vi "RX OOB Test Cases.vi"() -> (0 "error out":errorcluster, 2 "status":string, 3 "pass":bool)   [LabVIEW 2021]
uses:
  OOB_Rx/CIFCoreOOB_Rx.lvclass/CIFCoreOOB_Rx.ctl
  CIFUtilities/CIFOutOfBand/CIFOutOfBand.lvclass/CIFOutOfBand.ctl
  OOB_Rx/Typedef/OOB Core Commands.ctl
  OOB_Rx/Typedef/Channel Connection Data.ctl
  OOB_Rx/Private/Command Settings.vi
  CIFUtilities/CIFOutOfBand/Accessors/Write Local OOB Data.vi
  CIFUtilities/CIFOutOfBand/Write OOB DVR.vi
  CIFUtilities/CIFOutOfBand/Utilities/Command to Bitwise Command.vi
  CIFUtilities/CIFOutOfBand/Read OOB DVR.vi
  OOB_Rx/Private/Read Payload.vi
  OOB_Rx/CIFCoreOOB_Rx.lvclass
  D:/dev/CIF-LVCore/src/CIFUtilities/CIFOutOfBand/CIFOutOfBand.lvclass
  CIFUtilities/CIFOutOfBand/Init OOB.vi
  <vilib>/addons/_JKI.lib/Serialization/JSON/Library/Unflatten From JSON String.vi
  <vilib>/addons/_JKI.lib/Serialization/JSON/JKI JSON Serialization.lvlib
  CIFUtilities/CIFOutOfBand/CIFOutOfBand.lvclass
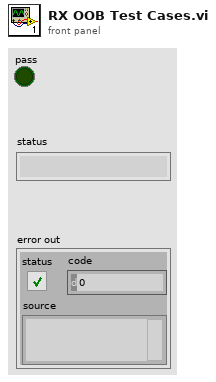
[diagram p1: front panel]
types:
  T1 = cluster{"Numeric":dbl, "Array":cluster{"Numeric":dbl, "String":string, "Boolean":bool}[], "string":string, "Null array":u8[]}
  T2 = typedef "CIFCoreOOB_Rx.lvclass/OOB Core Commands.ctl" = enum8{"Start", "Pause", "Stop", "RefreshStats", "UpdateConfig", "Connect Channel"}
  T3 = typedef "CIFCoreOOB_Rx.lvclass/Channel Connection Data.ctl" = cluster{"Publisher Name":string, "Subscriber Name":string, "Connection Data":variant}
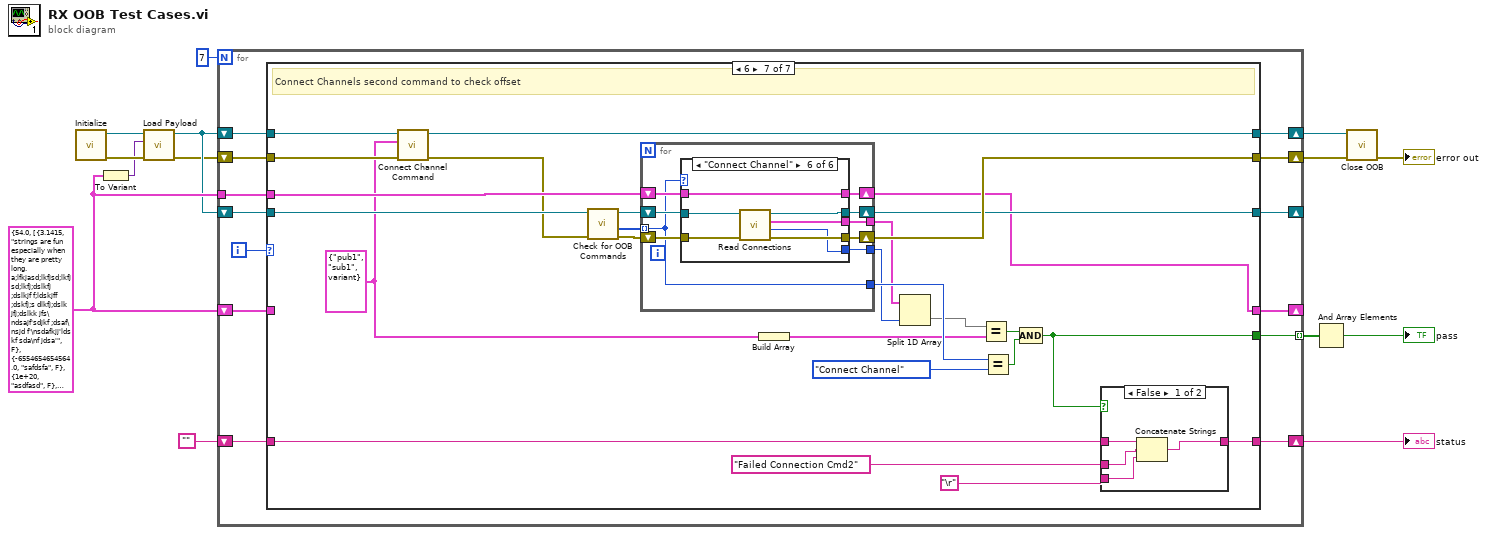
[diagram p0: block diagram]
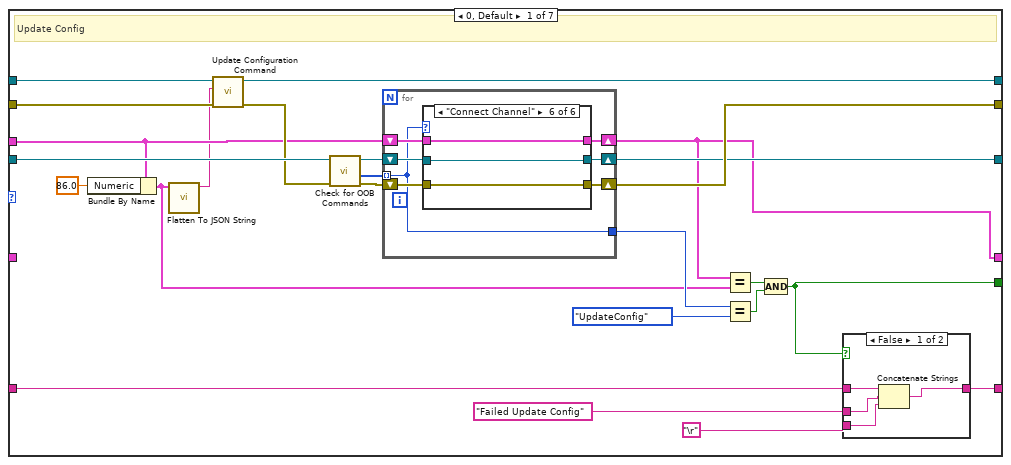
[diagram p2: hidden frame]
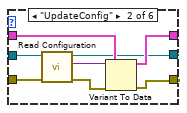
[diagram p4: hidden frame]
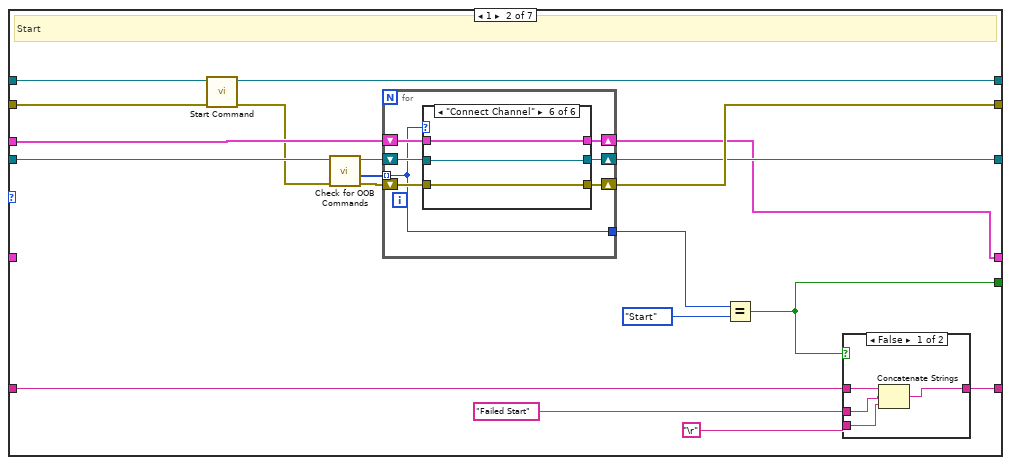
[diagram p9: hidden frame]
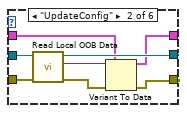
[diagram p11: hidden frame]
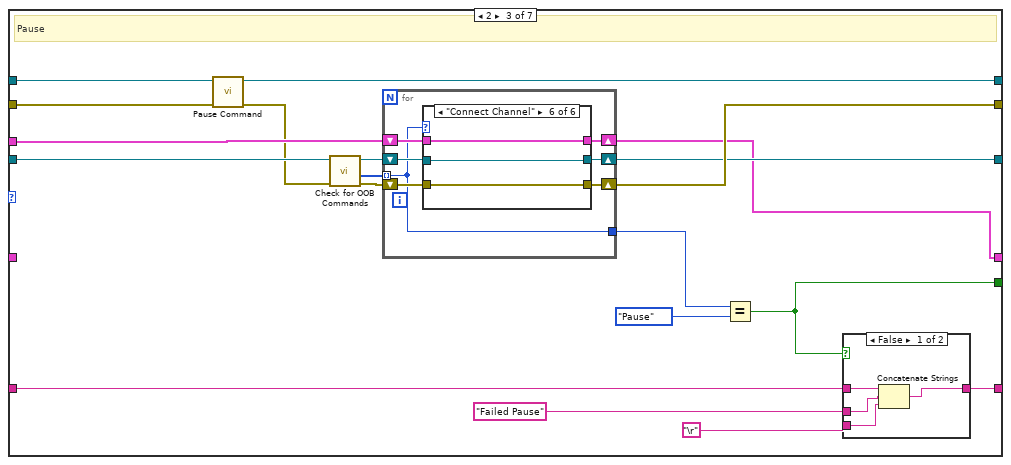
[diagram p16: hidden frame]
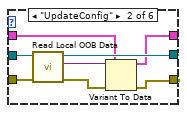
[diagram p18: hidden frame]
diagram:
  w14 = T1 {"Numeric"=54.0, "Array"=[{"Numeric"=3.1415, "String"="strings are fun especially when they are pretty long. a;lfkjasd;lkfjsd;lkfjsd;lkfj;dslkfj ;dslkjf f;ldskjff ;dskfj;s dlkfj;dslk jfj;dslkk jfs\ndsajf'sdjkf ;dsaf\nsjd f'\nsdafkjj'lds kf sda\nf jdsa'", "Boolean"=FALSE}, {"Numeric"=-6554654654564.0, "String"="safdsfa", "Boolean"=FALSE}, {"Numeric"=1e+20, "String"="asdfasd", "Boolean"=FALSE}, {"Numeric"=2.0, "String"="afd", "Boolean"=TRUE}, {"Numeric"=12.34, "String"="data", "Boolean"=FALSE}], "string"="strings", "Null array"=[0]} ("Test Config")
  n1 = call "Initialize.vi"() -> ("error out"=w7:errorcluster, "CoreOOB_Rx out"=w6:refnum<class "CIFCoreOOB_Rx.lvclass">)  [unwired: 10 in]
  n2 = To Variant(anything=w14) -> (Variant=w3:variant)
  n3 = call "Load Payload.vi"("error in (no error)"=w7, "Configuration Payload"=w3, "CoreOOB_Rx in"=w6) -> ("error out"=w4:errorcluster, "CoreOOB_Rx out"=w5:refnum<class "CIFCoreOOB_Rx.lvclass">)  [unwired: 7 in]
  n4 = for {
    N: 7 -> [_]
    tunnel: [w27] -> w11 mode=indexing
    tunnel: w14 -> [w25]
    shift-right: [w23] -> w12
    shift-left: w4 -> [w26]
    shift-right: [w21] -> w13
    shift-left: w5 -> [w24]
    shift-right: [w19] -> _
    shift-left: w5 -> [w20]
    shift-right: [w18] -> _
    shift-left: w14 -> [w17]
    shift-right: [w15] -> w8
    shift-left: "" -> [w16]
    i -> [w22]
    n5 = case shown="6" w22 {
      tunnel: [w39 w87 w141 w199 w253 w303 w370] -> w27
      tunnel: w26 -> [w34 w96 w144 w197 w251 w313 w380]
      tunnel: w25 -> [w32 w105 w159 w213 w267 w328 w395]
      tunnel: w24 -> [w36 w97 w145 w198 w252 w314 w381]
      tunnel: [w51 w104 w158 w212 w266 w327 w394] -> w23
      tunnel: [w35 w95 w142 w195 w249 w311 w378] -> w21
      tunnel: w20 -> [w45 w94 w151 w205 w259 w320 w387]
      tunnel: [w50 w103 w157 w211 w265 w326 w393] -> w19
      tunnel: [w28 w102 w156 w210 w264 w325 w392] -> w18
      tunnel: w17 -> [_ _ _ _ _ _ _]
      tunnel: w16 -> [w49 w101 w155 w209 w263 w324 w391]
      tunnel: [w48 w100 w154 w208 w262 w323 w390] -> w15
      frame 0, Default {
        # "Update Config"
        n6 = Bundle By Name(cluster=w32, "Numeric"=86.0) -> (w29:T1)
        n7 = call <vilib>:"Flatten To JSON String.vi"("Variant"=w29) -> ("JSON String"=w30:string)  [unwired: 9 in, 1 out]
        n8 = call "Update Configuration Command.vi"("error in"=w34, "Config JSON"=w30, "CoreOOB_Rx in"=w36) -> ("error out"=w33:errorcluster, "CoreOOB_Rx out"=w35:refnum<class "CIFCoreOOB_Rx.lvclass">)  [unwired: 7 in]
        n9 = call "Check for OOB Commands.vi"("error in (no error)"=w33, "CoreOOB_Rx in"=w45) -> ("error out"=w44:errorcluster, "Commands"=w42:T2[], "CoreOOB_Rx out"=w43:refnum<class "CIFCoreOOB_Rx.lvclass">)  [unwired: 6 in, 1 out]
        n10 = for {
          tunnel: w42 -> [w52] mode=indexing
          shift-right: [w53] -> w28
          shift-left: w32 -> [w58]
          shift-right: [w57] -> w51
          shift-left: w44 -> [w55]
          shift-right: [w56] -> w50
          shift-left: w43 -> [w54]
          tunnel: [w52] -> w38
          n11 = case shown="\"Connect Channel\"" w52 {
            tunnel: w54 -> [w60 w65 w71 w74 w77 w80]
            tunnel: w55 -> [w59 w66 w70 w73 w78 w81]
            tunnel: [w60 w64 w71 w74 w77 w80] -> w56
            tunnel: w58 -> [w61 w69 w72 w75 w76 w79]
            tunnel: [w59 w68 w70 w73 w78 w81] -> w57
            tunnel: [w61 w67 w72 w75 w76 w79] -> w53
            frame "Start" {
            }
            frame "UpdateConfig" {
              n12 = call "Read Configuration.vi"("error in"=w66, "CoreOOB_Rx in"=w65) -> ("error out"=w62:errorcluster, "Configuration Data"=w63:variant, "CoreOOB_Rx out"=w64:refnum<class "CIFCoreOOB_Rx.lvclass">)  [unwired: 7 in]
              n13 = Variant To Data(error in=w62, type=w69, Variant=w63) -> (data=w67:T1, error out=w68:errorcluster)
            }
            frame "Pause" {
            }
            frame "Stop" {
            }
            frame "RefreshStats" {
            }
            frame "Connect Channel" {
            }
          }
        }
        n14 = Equal?(x=w28, y=w29) -> (x = y?=w41:bool)
        n15 = Equal?(x=w38, y=OOB_Core_Commands."UpdateConfig") -> (x = y?=w40:bool)
        n16 = Compound Arithmetic op=AND(w41, w40) -> (w39:bool)
        n17 = case shown="False" w39 {
          tunnel: w49 -> [w85 w86]
          tunnel: [w82 w86] -> w48
          tunnel: "Failed Update Config" -> [w84 _]
          tunnel: "\r" -> [w83 _]
          frame False {
            n18 = Concatenate Strings(w85, w84, w83) -> (w82:string)
          }
          frame True {
          }
        }
      }
      frame 1 {
        # "Start"
        n19 = call "Start Command.vi"("error in"=w96, "CoreOOB_Rx in"=w97) -> ("error out"=w93:errorcluster, "CoreOOB_Rx out"=w95:refnum<class "CIFCoreOOB_Rx.lvclass">)  [unwired: 8 in]
        n20 = call "Check for OOB Commands.vi"("error in (no error)"=w93, "CoreOOB_Rx in"=w94) -> ("error out"=w92:errorcluster, "Commands"=w90:T2[], "CoreOOB_Rx out"=w91:refnum<class "CIFCoreOOB_Rx.lvclass">)  [unwired: 6 in, 1 out]
        n21 = for {
          tunnel: w90 -> [w106] mode=indexing
          shift-right: [w107] -> w102
          shift-left: w105 -> [w112]
          shift-right: [w111] -> w104
          shift-left: w92 -> [w109]
          shift-right: [w110] -> w103
          shift-left: w91 -> [w108]
          tunnel: [w106] -> w89
          n22 = case shown="\"Connect Channel\"" w106 {
            tunnel: w108 -> [w113 w123 w125 w128 w131 w134]
            tunnel: w109 -> [w114 w122 w124 w127 w132 w135]
            tunnel: [w113 w120 w125 w128 w131 w134] -> w110
            tunnel: w112 -> [w115 w118 w126 w129 w130 w133]
            tunnel: [w114 w117 w124 w127 w132 w135] -> w111
            tunnel: [w115 w116 w126 w129 w130 w133] -> w107
            frame "Start" {
            }
            frame "UpdateConfig" {
              n23 = call "Read Local OOB Data.vi"("error in"=w122, "OOB in"=w123) -> ("error out"=w121:errorcluster, "Local OOB Data"=w119:variant, "OOB out"=w120:refnum<class "CIFCoreOOB_Rx.lvclass">)  [unwired: 7 in]
              n24 = Variant To Data(error in=w121, type=w118, Variant=w119) -> (data=w116:T1, error out=w117:errorcluster)
            }
            frame "Pause" {
            }
            frame "Stop" {
            }
            frame "RefreshStats" {
            }
            frame "Connect Channel" {
            }
          }
        }
        n25 = Equal?(x=w89, y=OOB_Core_Commands."Start") -> (x = y?=w87:bool)
        n26 = case shown="False" w87 {
          tunnel: w101 -> [w139 w140]
          tunnel: [w136 w140] -> w100
          tunnel: "Failed Start" -> [w138 _]
          tunnel: "\r" -> [w137 _]
          frame False {
            n27 = Concatenate Strings(w139, w138, w137) -> (w136:string)
          }
          frame True {
          }
        }
      }
      frame 2 {
        # "Pause"
        n28 = call "Pause Command.vi"("error in"=w144, "CoreOOB_Rx in"=w145) -> ("error out"=w143:errorcluster, "CoreOOB_Rx out"=w142:refnum<class "CIFCoreOOB_Rx.lvclass">)  [unwired: 8 in]
        n29 = call "Check for OOB Commands.vi"("error in (no error)"=w143, "CoreOOB_Rx in"=w151) -> ("error out"=w150:errorcluster, "Commands"=w148:T2[], "CoreOOB_Rx out"=w149:refnum<class "CIFCoreOOB_Rx.lvclass">)  [unwired: 6 in, 1 out]
        n30 = for {
          tunnel: w148 -> [w160] mode=indexing
          shift-right: [w161] -> w156
          shift-left: w159 -> [w166]
          shift-right: [w165] -> w158
          shift-left: w150 -> [w163]
          shift-right: [w164] -> w157
          shift-left: w149 -> [w162]
          tunnel: [w160] -> w147
          n31 = case shown="\"Connect Channel\"" w160 {
            tunnel: w162 -> [w168 w177 w179 w182 w185 w188]
            tunnel: w163 -> [w167 w176 w178 w181 w186 w189]
            tunnel: [w168 w174 w179 w182 w185 w188] -> w164
            tunnel: w166 -> [w169 w172 w180 w183 w184 w187]
            tunnel: [w167 w171 w178 w181 w186 w189] -> w165
            tunnel: [w169 w170 w180 w183 w184 w187] -> w161
            frame "Start" {
            }
            frame "UpdateConfig" {
              n32 = call "Read Local OOB Data.vi"("error in"=w176, "OOB in"=w177) -> ("error out"=w175:errorcluster, "Local OOB Data"=w173:variant, "OOB out"=w174:refnum<class "CIFCoreOOB_Rx.lvclass">)  [unwired: 7 in]
              n33 = Variant To Data(error in=w175, type=w172, Variant=w173) -> (data=w170:T1, error out=w171:errorcluster)
            }
            frame "Pause" {
            }
            frame "Stop" {
            }
            frame "RefreshStats" {
            }
            frame "Connect Channel" {
            }
          }
        }
        n34 = Equal?(x=w147, y=OOB_Core_Commands."Pause") -> (x = y?=w141:bool)
        n35 = case shown="False" w141 {
          tunnel: w155 -> [w193 w194]
          tunnel: [w190 w194] -> w154
          tunnel: "Failed Pause" -> [w192 _]
          tunnel: "\r" -> [w191 _]
          frame False {
            n36 = Concatenate Strings(w193, w192, w191) -> (w190:string)
          }
          frame True {
          }
        }
      }
      frame 3 {
        # "Stop"
        n37 = call "Stop Command.vi"("error in"=w197, "CoreOOB_Rx in"=w198) -> ("error out"=w196:errorcluster, "CoreOOB_Rx out"=w195:refnum<class "CIFCoreOOB_Rx.lvclass">)  [unwired: 8 in]
        n38 = call "Check for OOB Commands.vi"("error in (no error)"=w196, "CoreOOB_Rx in"=w205) -> ("error out"=w204:errorcluster, "Commands"=w202:T2[], "CoreOOB_Rx out"=w203:refnum<class "CIFCoreOOB_Rx.lvclass">)  [unwired: 6 in, 1 out]
        n39 = for {
          tunnel: w202 -> [w214] mode=indexing
          shift-right: [w215] -> w210
          shift-left: w213 -> [w220]
          shift-right: [w219] -> w212
          shift-left: w204 -> [w217]
          shift-right: [w218] -> w211
          shift-left: w203 -> [w216]
          tunnel: [w214] -> w201
          n40 = case shown="\"Connect Channel\"" w214 {
            tunnel: w216 -> [w222 w231 w233 w236 w239 w242]
            tunnel: w217 -> [w221 w230 w232 w235 w240 w243]
            tunnel: [w222 w228 w233 w236 w239 w242] -> w218
            tunnel: w220 -> [w223 w226 w234 w237 w238 w241]
            tunnel: [w221 w225 w232 w235 w240 w243] -> w219
            tunnel: [w223 w224 w234 w237 w238 w241] -> w215
            frame "Start" {
            }
            frame "UpdateConfig" {
              n41 = call "Read Local OOB Data.vi"("error in"=w230, "OOB in"=w231) -> ("error out"=w229:errorcluster, "Local OOB Data"=w227:variant, "OOB out"=w228:refnum<class "CIFCoreOOB_Rx.lvclass">)  [unwired: 7 in]
              n42 = Variant To Data(error in=w229, type=w226, Variant=w227) -> (data=w224:T1, error out=w225:errorcluster)
            }
            frame "Pause" {
            }
            frame "Stop" {
            }
            frame "RefreshStats" {
            }
            frame "Connect Channel" {
            }
          }
        }
        n43 = Equal?(x=w201, y=OOB_Core_Commands."Stop") -> (x = y?=w199:bool)
        n44 = case shown="False" w199 {
          tunnel: w209 -> [w247 w248]
          tunnel: [w244 w248] -> w208
          tunnel: "Failed Stop" -> [w246 _]
          tunnel: "\r" -> [w245 _]
          frame False {
            n45 = Concatenate Strings(w247, w246, w245) -> (w244:string)
          }
          frame True {
          }
        }
      }
      frame 4 {
        # "Refresh"
        n46 = call "Refresh Stats Command.vi"("error in"=w251, "CoreOOB_Rx in"=w252) -> ("error out"=w250:errorcluster, "CoreOOB_Rx out"=w249:refnum<class "CIFCoreOOB_Rx.lvclass">)  [unwired: 8 in]
        n47 = call "Check for OOB Commands.vi"("error in (no error)"=w250, "CoreOOB_Rx in"=w259) -> ("error out"=w258:errorcluster, "Commands"=w256:T2[], "CoreOOB_Rx out"=w257:refnum<class "CIFCoreOOB_Rx.lvclass">)  [unwired: 6 in, 1 out]
        n48 = for {
          tunnel: w256 -> [w268] mode=indexing
          shift-right: [w269] -> w264
          shift-left: w267 -> [w274]
          shift-right: [w273] -> w266
          shift-left: w258 -> [w271]
          shift-right: [w272] -> w265
          shift-left: w257 -> [w270]
          tunnel: [w268] -> w255
          n49 = case shown="\"Connect Channel\"" w268 {
            tunnel: w270 -> [w276 w285 w287 w290 w293 w296]
            tunnel: w271 -> [w275 w284 w286 w289 w294 w297]
            tunnel: [w276 w282 w287 w290 w293 w296] -> w272
            tunnel: w274 -> [w277 w280 w288 w291 w292 w295]
            tunnel: [w275 w279 w286 w289 w294 w297] -> w273
            tunnel: [w277 w278 w288 w291 w292 w295] -> w269
            frame "Start" {
            }
            frame "UpdateConfig" {
              n50 = call "Read Local OOB Data.vi"("error in"=w284, "OOB in"=w285) -> ("error out"=w283:errorcluster, "Local OOB Data"=w281:variant, "OOB out"=w282:refnum<class "CIFCoreOOB_Rx.lvclass">)  [unwired: 7 in]
              n51 = Variant To Data(error in=w283, type=w280, Variant=w281) -> (data=w278:T1, error out=w279:errorcluster)
            }
            frame "Pause" {
            }
            frame "Stop" {
            }
            frame "RefreshStats" {
            }
            frame "Connect Channel" {
            }
          }
        }
        n52 = Equal?(x=w255, y=OOB_Core_Commands."RefreshStats") -> (x = y?=w253:bool)
        n53 = case shown="False" w253 {
          tunnel: w263 -> [w301 w302]
          tunnel: [w298 w302] -> w262
          tunnel: "Failed Refresh" -> [w300 _]
          tunnel: "\r" -> [w299 _]
          frame False {
            n54 = Concatenate Strings(w301, w300, w299) -> (w298:string)
          }
          frame True {
          }
        }
      }
      frame 5 {
        w307 = T3 {"Publisher Name"="pub", "Subscriber Name"="sub", "Connection Data"=variant} ("Channel Connection Data")
        # "Connect Channels"
        n55 = call "Connect Channel Command.vi"("error in"=w313, "Channel Connection Data"=w307, "CoreOOB_Rx in"=w314) -> ("error out"=w312:errorcluster, "CoreOOB_Rx out"=w311:refnum<class "CIFCoreOOB_Rx.lvclass">)  [unwired: 7 in]
        n56 = call "Check for OOB Commands.vi"("error in (no error)"=w312, "CoreOOB_Rx in"=w320) -> ("error out"=w319:errorcluster, "Commands"=w317:T2[], "CoreOOB_Rx out"=w318:refnum<class "CIFCoreOOB_Rx.lvclass">)  [unwired: 6 in, 1 out]
        n57 = for {
          tunnel: w317 -> [w331] mode=indexing
          shift-right: [w332] -> w325
          shift-left: w328 -> [w337]
          shift-right: [w336] -> w327
          shift-left: w319 -> [w334]
          shift-right: [w335] -> w326
          shift-left: w318 -> [w333]
          tunnel: [w331] -> w316
          tunnel: [w330] -> w310
          tunnel: [w329] -> w309
          n58 = case shown="\"Connect Channel\"" w331 {
            tunnel: w333 -> [w339 w348 w350 w353 w356 w363]
            tunnel: w334 -> [w338 w347 w349 w352 w357 w362]
            tunnel: [w339 w345 w350 w353 w356 w361] -> w335
            tunnel: w337 -> [w340 w343 w351 w354 w355 w364]
            tunnel: [w338 w342 w349 w352 w357 w360] -> w336
            tunnel: [w340 w341 w351 w354 w355 w364] -> w332
            tunnel: [_ _ _ _ _ w359] -> w330
            tunnel: [_ _ _ _ _ w358] -> w329
            frame "Start" {
            }
            frame "UpdateConfig" {
              n59 = call "Read Local OOB Data.vi"("error in"=w347, "OOB in"=w348) -> ("error out"=w346:errorcluster, "Local OOB Data"=w344:variant, "OOB out"=w345:refnum<class "CIFCoreOOB_Rx.lvclass">)  [unwired: 7 in]
              n60 = Variant To Data(error in=w346, type=w343, Variant=w344) -> (data=w341:T1, error out=w342:errorcluster)
            }
            frame "Pause" {
            }
            frame "Stop" {
            }
            frame "RefreshStats" {
            }
            frame "Connect Channel" {
              n61 = call "Read Connections.vi"("error in"=w362, "CoreOOB_Rx in"=w363) -> ("error out"=w360:errorcluster, "Offset"=w358:i32, "Connections"=w359:T3[], "CoreOOB_Rx out"=w361:refnum<class "CIFCoreOOB_Rx.lvclass">)  [unwired: 6 in]
            }
          }
        }
        n62 = Build Array(w307) -> (w306:T3[])
        n63 = Split 1D Array(array=w310, index=w309) -> (second subarray=w308:T3[])  [unwired: 1 out]
        n64 = Equal?(x=w308, y=w306) -> (x = y?=w305:bool)
        n65 = Equal?(x=w316, y=OOB_Core_Commands."Connect Channel") -> (x = y?=w304:bool)
        n66 = Compound Arithmetic op=AND(w305, w304) -> (w303:bool)
        n67 = case shown="False" w303 {
          tunnel: w324 -> [w368 w369]
          tunnel: [w365 w369] -> w323
          tunnel: "Failed Connection Cmd1" -> [w367 _]
          tunnel: "\r" -> [w366 _]
          frame False {
            n68 = Concatenate Strings(w368, w367, w366) -> (w365:string)
          }
          frame True {
          }
        }
      }
      frame 6 {
        w374 = T3 {"Publisher Name"="pub1", "Subscriber Name"="sub1", "Connection Data"=variant} ("Channel Connection Data")
        # "Connect Channels second command to check offset"
        n69 = call "Connect Channel Command.vi"("error in"=w380, "Channel Connection Data"=w374, "CoreOOB_Rx in"=w381) -> ("error out"=w379:errorcluster, "CoreOOB_Rx out"=w378:refnum<class "CIFCoreOOB_Rx.lvclass">)  [unwired: 7 in]
        n70 = call "Check for OOB Commands.vi"("error in (no error)"=w379, "CoreOOB_Rx in"=w387) -> ("error out"=w386:errorcluster, "Commands"=w384:T2[], "CoreOOB_Rx out"=w385:refnum<class "CIFCoreOOB_Rx.lvclass">)  [unwired: 6 in, 1 out]
        n71 = for {
          tunnel: w384 -> [w398] mode=indexing
          shift-right: [w399] -> w392
          shift-left: w395 -> [w404]
          shift-right: [w403] -> w394
          shift-left: w386 -> [w401]
          shift-right: [w402] -> w393
          shift-left: w385 -> [w400]
          tunnel: [w398] -> w383
          tunnel: [w397] -> w377
          tunnel: [w396] -> w376
          n72 = case shown="\"Connect Channel\"" w398 {
            tunnel: w400 -> [w406 w415 w417 w420 w423 w430]
            tunnel: w401 -> [w405 w414 w416 w419 w424 w429]
            tunnel: [w406 w412 w417 w420 w423 w428] -> w402
            tunnel: w404 -> [w407 w410 w418 w421 w422 w431]
            tunnel: [w405 w409 w416 w419 w424 w427] -> w403
            tunnel: [w407 w408 w418 w421 w422 w431] -> w399
            tunnel: [_ _ _ _ _ w426] -> w397
            tunnel: [_ _ _ _ _ w425] -> w396
            frame "Start" {
            }
            frame "UpdateConfig" {
              n73 = call "Read Local OOB Data.vi"("error in"=w414, "OOB in"=w415) -> ("error out"=w413:errorcluster, "Local OOB Data"=w411:variant, "OOB out"=w412:refnum<class "CIFCoreOOB_Rx.lvclass">)  [unwired: 7 in]
              n74 = Variant To Data(error in=w413, type=w410, Variant=w411) -> (data=w408:T1, error out=w409:errorcluster)
            }
            frame "Pause" {
            }
            frame "Stop" {
            }
            frame "RefreshStats" {
            }
            frame "Connect Channel" {
              n75 = call "Read Connections.vi"("error in"=w429, "CoreOOB_Rx in"=w430) -> ("error out"=w427:errorcluster, "Offset"=w425:i32, "Connections"=w426:T3[], "CoreOOB_Rx out"=w428:refnum<class "CIFCoreOOB_Rx.lvclass">)  [unwired: 6 in]
            }
          }
        }
        n76 = Build Array(w374) -> (w373:T3[])
        n77 = Split 1D Array(array=w377, index=w376) -> (second subarray=w375:T3[])  [unwired: 1 out]
        n78 = Equal?(x=w375, y=w373) -> (x = y?=w372:bool)
        n79 = Equal?(x=w383, y=OOB_Core_Commands."Connect Channel") -> (x = y?=w371:bool)
        n80 = Compound Arithmetic op=AND(w372, w371) -> (w370:bool)
        n81 = case shown="False" w370 {
          tunnel: w391 -> [w435 w436]
          tunnel: [w432 w436] -> w390
          tunnel: "Failed Connection Cmd2" -> [w434 _]
          tunnel: "\r" -> [w433 _]
          frame False {
            n82 = Concatenate Strings(w435, w434, w433) -> (w432:string)
          }
          frame True {
          }
        }
      }
    }
  }
  "status" <- w8
  n83 = And Array Elements(Boolean array=w11) -> (logical AND=→"pass":bool)
  n84 = call "Close OOB.vi"("error in"=w12, "OOB in"=w13) -> ("error out"=→"error out":errorcluster)  [unwired: 9 in]
